vi "Verify String Input.vi"(8 "error in (no error)":errorcluster, 10 "Error Message":string, 11 "Input":string) -> (0 "error out":errorcluster, 3 "Output":string)   [LabVIEW 2024, in "Sift Client.lvlib"]
doc: "Verifies that input string is not empty. Otherwise and error is raised."
uses:
  <vilib>/Utility/error.llb/Trim Whitespace One-Sided.vi
  Sift Client.lvlib
  <userlib>/_OpenG.lib/error/error.llb/openg_error.lvlib
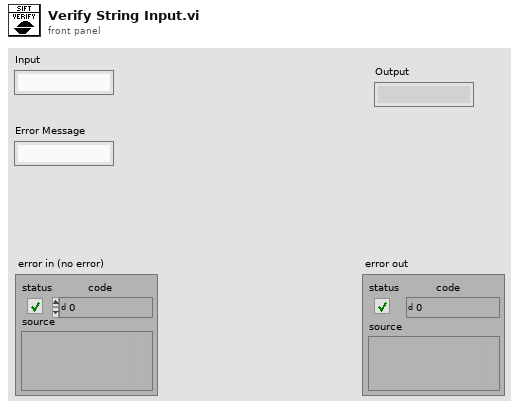
[diagram p1: front panel]
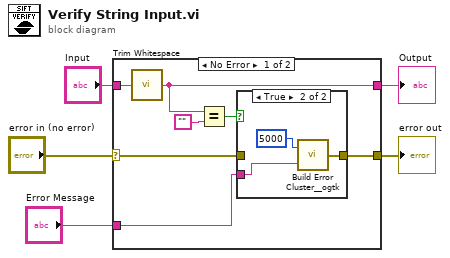
[diagram p0: block diagram]
diagram:
  n1 = case shown="No Error" "error in (no error)" {
    selector: "error in (no error)" -> [w6 w18]
    tunnel: [w7 w18] -> w4
    tunnel: "Error Message" -> [w8 _]
    tunnel: "Input" -> [w12 w17]
    tunnel: [w10 w17] -> w1
    frame No Error {
      n2 = call <vilib>:"Trim Whitespace.vi"("string"=w12) -> ("trimmed string"=w10:string)  [unwired: 1 in]
      n3 = Equal?(x=w10, y="") -> (x = y?=w9:bool)
      n4 = case shown="True" w9 {
        tunnel: w8 -> [_ w16]
        tunnel: [w13 w14] -> w7
        tunnel: w6 -> [w13 _]
        frame False {
        }
        frame True {
          n5 = call <userlib>:"Build Error Cluster__ogtk.vi"("String to Prepend to source (\"\")"=w16, "code"=5000) -> ("error out"=w14:errorcluster)
        }
      }
    }
    frame Error {
    }
  }
  "error out" <- w4
  "Output" <- w1
